vi "write_param.vi"   [LabVIEW 2012]
uses:
  FT_HMI.llb/GLOBAL_PUMPS_PARAMS.vi
  FT_HMI.llb/GLOBAL_GEN.vi
  ADS.llb/Global DIOs.vi
types:
  T1 = cluster{"VAC":cluster{"ENABLE":bool, "PUMPING_TIME [ms]":dbl, "MEASUREMENT_TIME [ms]":dbl, "PRESSURE_LIMIT [bar]":sgl}, "Q1":cluster{"ENABLE":bool, "PUMPING_TIME  [ms]":dbl, "MEASUREMENT_TIME  [ms]":sgl, "FLOW_TARGET  [ml/min]":sgl, "FLOW_LIMIT_UP  [ml/min]":sgl, "FLOW_LIMIT_DOWN [ml/min]":sgl, "PRESSURE_TARGET [bar]":sgl, "PRESSURE_LIMIT_UP [bar]":sgl, "PRESSURE_LIMIT_DOWN [bar]":sgl, "MAX_FLOW":bool}, "Q2":cluster{"ENABLE":bool, "PUMPING_TIME [ms]":dbl, "MEASUREMENT_TIME [ms]":dbl, "FLOW_TARGET [ml/min]":sgl, "FLOW_LIMIT_UP [ml/min]":sgl, "FLOW_LIMIT_DOWN [ml/min]":sgl, "PRESSURE_TARGET [bar]":sgl, "PRESSURE_LIMIT_UP [bar]":sgl, "PRESSURE_LIMIT_DOWN [bar]":sgl, "MAX_FLOW":bool}, "PMAX":cluster{"ENABLE":bool, "PUMPING_TIME [ms]":dbl, "MEASUREMENT_TIME [ms]":dbl, "PRESSURE_LIMIT [bar]":sgl, "PRESSURE_LOOSE_TIME [ms]":sgl}, "PRINT":cluster{"ENABLE":bool}, "SUPPLY":cluster{"VOLTAGE [V]":dbl, "FREQUENCY [Hz]":dbl}}
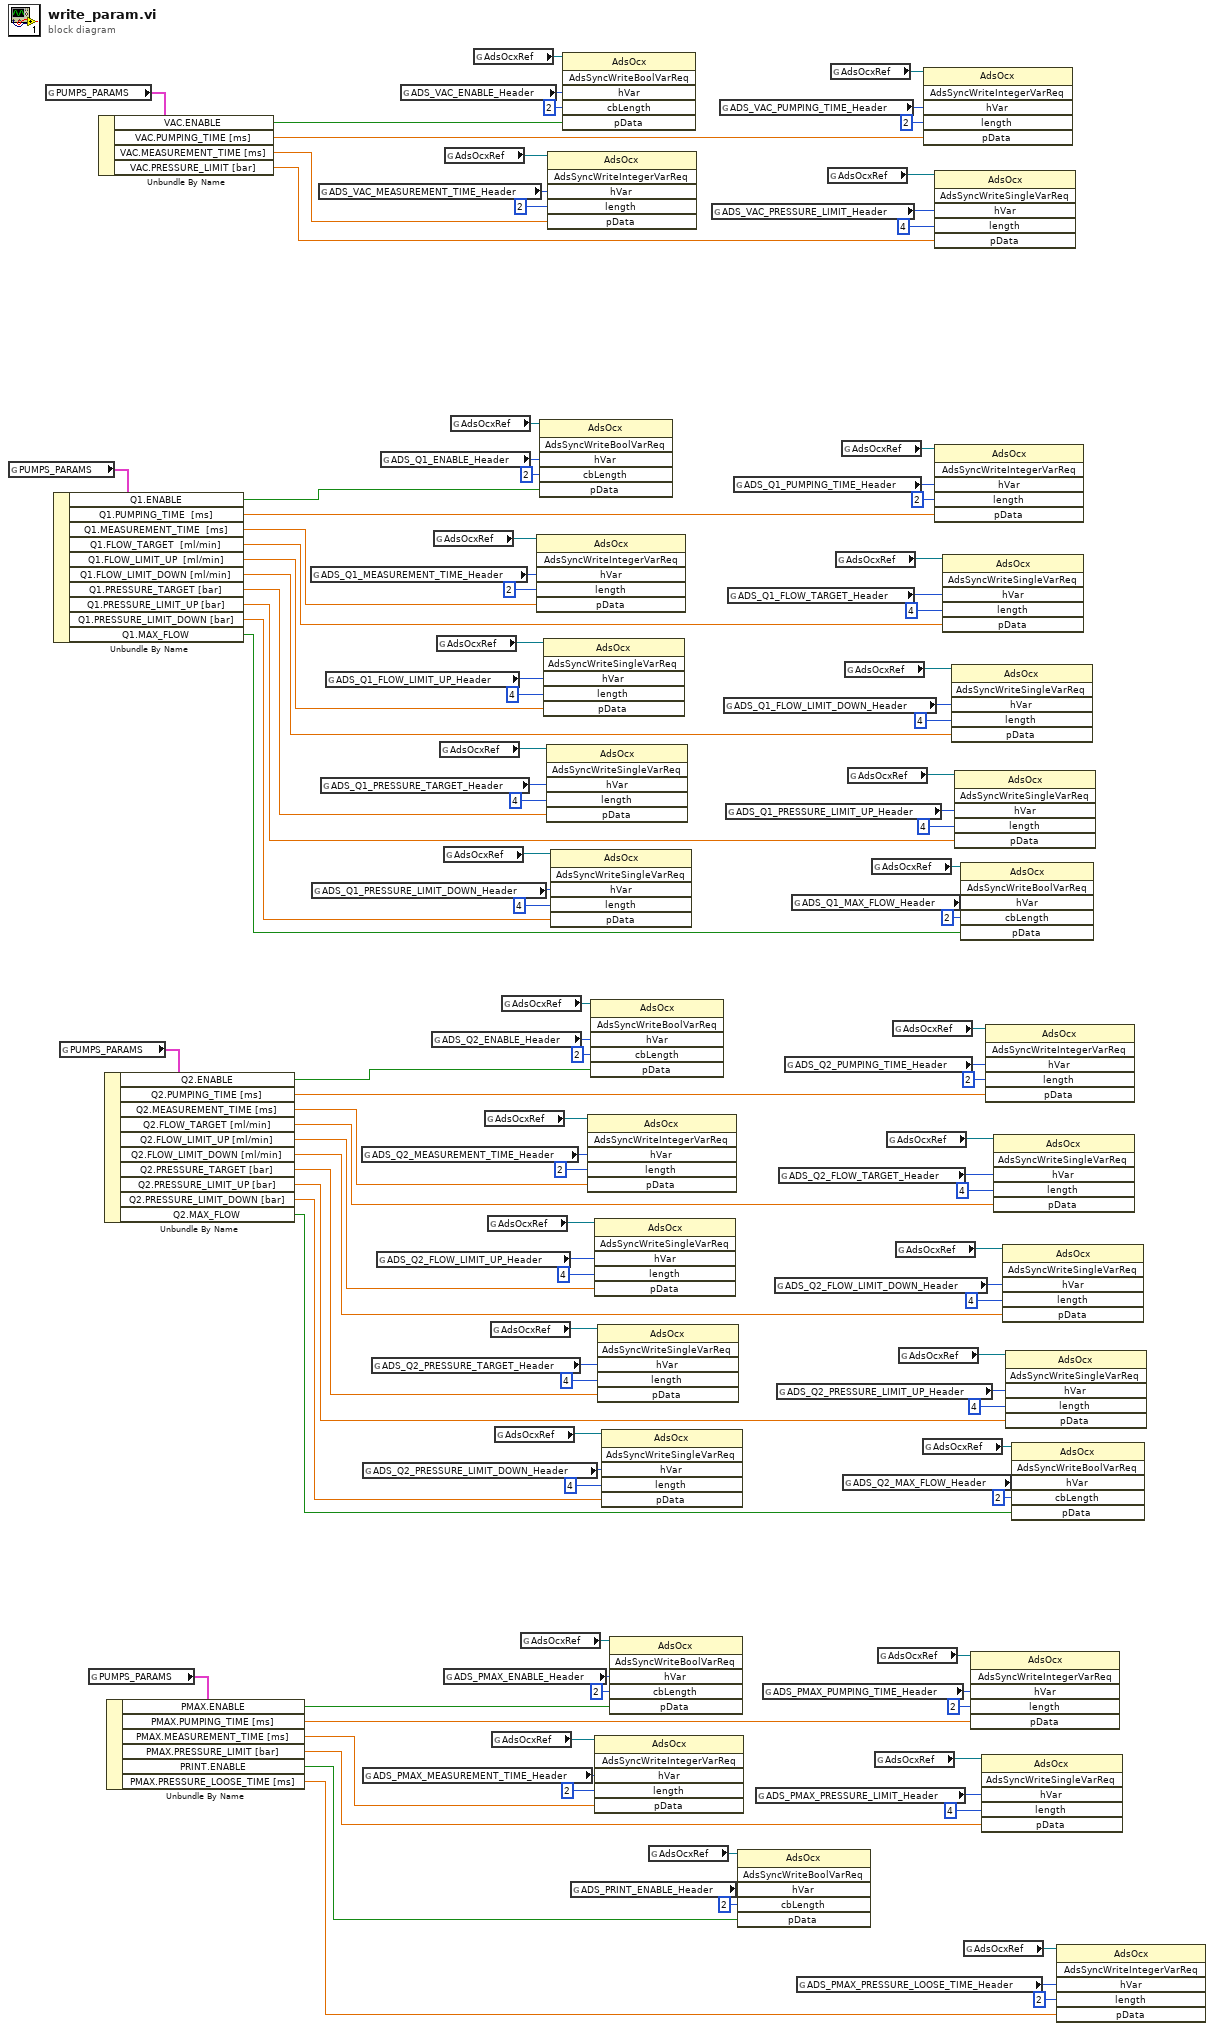
[diagram p0: block diagram]
diagram:
  n1 = global read "GLOBAL_PUMPS_PARAMS.vi" "PUMPS_PARAMS"() -> (w107:T1)
  n2 = global read "GLOBAL_PUMPS_PARAMS.vi" "PUMPS_PARAMS"() -> (w124:T1)
  n3 = Unbundle By Name(w107) -> ("Q1.ENABLE"=w103:bool, "Q1.PUMPING_TIME  [ms]"=w99:dbl, "Q1.MEASUREMENT_TIME  [ms]"=w95:sgl, "Q1.FLOW_TARGET  [ml/min]"=w91:sgl, "Q1.FLOW_LIMIT_UP  [ml/min]"=w83:sgl, "Q1.FLOW_LIMIT_DOWN [ml/min]"=w84:sgl, "Q1.PRESSURE_TARGET [bar]"=w76:sgl, "Q1.PRESSURE_LIMIT_UP [bar]"=w75:sgl, "Q1.PRESSURE_LIMIT_DOWN [bar]"=w71:sgl, "Q1.MAX_FLOW"=w67:bool)
  n4 = global read "GLOBAL_PUMPS_PARAMS.vi" "PUMPS_PARAMS"() -> (w66:T1)
  n5 = global read "GLOBAL_PUMPS_PARAMS.vi" "PUMPS_PARAMS"() -> (w25:T1)
  n6 = Unbundle By Name(w124) -> ("VAC.ENABLE"=w120:bool, "VAC.PUMPING_TIME [ms]"=w116:dbl, "VAC.MEASUREMENT_TIME [ms]"=w112:dbl, "VAC.PRESSURE_LIMIT [bar]"=w108:sgl)
  n7 = Unbundle By Name(w66) -> ("Q2.ENABLE"=w62:bool, "Q2.PUMPING_TIME [ms]"=w58:dbl, "Q2.MEASUREMENT_TIME [ms]"=w54:dbl, "Q2.FLOW_TARGET [ml/min]"=w50:sgl, "Q2.FLOW_LIMIT_UP [ml/min]"=w42:sgl, "Q2.FLOW_LIMIT_DOWN [ml/min]"=w43:sgl, "Q2.PRESSURE_TARGET [bar]"=w35:sgl, "Q2.PRESSURE_LIMIT_UP [bar]"=w34:sgl, "Q2.PRESSURE_LIMIT_DOWN [bar]"=w30:sgl, "Q2.MAX_FLOW"=w26:bool)
  n8 = Unbundle By Name(w25) -> ("PMAX.ENABLE"=w21:bool, "PMAX.PUMPING_TIME [ms]"=w17:dbl, "PMAX.MEASUREMENT_TIME [ms]"=w13:dbl, "PMAX.PRESSURE_LIMIT [bar]"=w9:sgl, "PRINT.ENABLE"=w5:bool, "PMAX.PRESSURE_LOOSE_TIME [ms]"=w1:sgl)
  n9 = global read "Global DIOs.vi" "ADS_Q1_MEASUREMENT_TIME_Header"() -> (w96:i32)
  n10 = global read "Global DIOs.vi" "ADS_Q1_PRESSURE_LIMIT_DOWN_Header"() -> (w72:i32)
  n11 = global read "Global DIOs.vi" "ADS_VAC_MEASUREMENT_TIME_Header"() -> (w113:i32)
  n12 = global read "Global DIOs.vi" "ADS_Q1_PRESSURE_TARGET_Header"() -> (w80:i32)
  n13 = global read "Global DIOs.vi" "ADS_Q1_FLOW_LIMIT_UP_Header"() -> (w88:i32)
  n14 = global read "Global DIOs.vi" "ADS_Q2_MEASUREMENT_TIME_Header"() -> (w55:i32)
  n15 = global read "Global DIOs.vi" "ADS_Q2_PRESSURE_LIMIT_DOWN_Header"() -> (w31:i32)
  n16 = global read "Global DIOs.vi" "ADS_PMAX_MEASUREMENT_TIME_Header"() -> (w14:i32)
  n17 = global read "Global DIOs.vi" "ADS_Q2_PRESSURE_TARGET_Header"() -> (w39:i32)
  n18 = global read "Global DIOs.vi" "ADS_Q2_FLOW_LIMIT_UP_Header"() -> (w47:i32)
  n19 = global read "Global DIOs.vi" "ADS_Q1_ENABLE_Header"() -> (w104:i32)
  n20 = global read "Global DIOs.vi" "ADS_VAC_ENABLE_Header"() -> (w121:i32)
  n21 = global read "Global DIOs.vi" "ADS_Q2_ENABLE_Header"() -> (w63:i32)
  n22 = global read "GLOBAL_GEN.vi" "AdsOcxRef"() -> (w97:refnum<k7>)
  n23 = global read "GLOBAL_GEN.vi" "AdsOcxRef"() -> (w89:refnum<k7>)
  n24 = global read "GLOBAL_GEN.vi" "AdsOcxRef"() -> (w81:refnum<k7>)
  n25 = global read "GLOBAL_GEN.vi" "AdsOcxRef"() -> (w73:refnum<k7>)
  n26 = global read "Global DIOs.vi" "ADS_PMAX_ENABLE_Header"() -> (w22:i32)
  n27 = global read "GLOBAL_GEN.vi" "AdsOcxRef"() -> (w114:refnum<k7>)
  n28 = global read "GLOBAL_GEN.vi" "AdsOcxRef"() -> (w105:refnum<k7>)
  n29 = global read "GLOBAL_GEN.vi" "AdsOcxRef"() -> (w122:refnum<k7>)
  n30 = global read "GLOBAL_GEN.vi" "AdsOcxRef"() -> (w56:refnum<k7>)
  n31 = global read "GLOBAL_GEN.vi" "AdsOcxRef"() -> (w48:refnum<k7>)
  n32 = global read "GLOBAL_GEN.vi" "AdsOcxRef"() -> (w40:refnum<k7>)
  n33 = global read "GLOBAL_GEN.vi" "AdsOcxRef"() -> (w15:refnum<k7>)
  n34 = global read "GLOBAL_GEN.vi" "AdsOcxRef"() -> (w32:refnum<k7>)
  n35 = global read "GLOBAL_GEN.vi" "AdsOcxRef"() -> (w64:refnum<k7>)
  n36 = global read "GLOBAL_GEN.vi" "AdsOcxRef"() -> (w23:refnum<k7>)
  n37 = invoke class="AdsOcx" method="AdsSyncWriteIntegerVarReq"(reference=w97, "hVar"=w96, "length"=2 ("phConnect"), "pData"=w95) -> ()  [unwired: 2 in, 6 out]
  n38 = invoke class="AdsOcx" method="AdsSyncWriteBoolVarReq"(reference=w105, "hVar"=w104, "cbLength"=2 ("phConnect"), "pData"=w103) -> ()  [unwired: 2 in, 6 out]
  n39 = invoke class="AdsOcx" method="AdsSyncWriteSingleVarReq"(reference=w89, "hVar"=w88, "length"=4 ("phConnect"), "pData"=w83) -> ()  [unwired: 2 in, 6 out]
  n40 = invoke class="AdsOcx" method="AdsSyncWriteSingleVarReq"(reference=w81, "hVar"=w80, "length"=4 ("phConnect"), "pData"=w76) -> ()  [unwired: 2 in, 6 out]
  n41 = invoke class="AdsOcx" method="AdsSyncWriteIntegerVarReq"(reference=w114, "hVar"=w113, "length"=2 ("phConnect"), "pData"=w112) -> ()  [unwired: 2 in, 6 out]
  n42 = invoke class="AdsOcx" method="AdsSyncWriteSingleVarReq"(reference=w73, "hVar"=w72, "length"=4 ("phConnect"), "pData"=w71) -> ()  [unwired: 2 in, 6 out]
  n43 = invoke class="AdsOcx" method="AdsSyncWriteBoolVarReq"(reference=w122, "hVar"=w121, "cbLength"=2 ("phConnect"), "pData"=w120) -> ()  [unwired: 2 in, 6 out]
  n44 = global read "Global DIOs.vi" "ADS_PRINT_ENABLE_Header"() -> (w6:i32)
  n45 = invoke class="AdsOcx" method="AdsSyncWriteIntegerVarReq"(reference=w56, "hVar"=w55, "length"=2 ("phConnect"), "pData"=w54) -> ()  [unwired: 2 in, 6 out]
  n46 = invoke class="AdsOcx" method="AdsSyncWriteBoolVarReq"(reference=w64, "hVar"=w63, "cbLength"=2 ("phConnect"), "pData"=w62) -> ()  [unwired: 2 in, 6 out]
  n47 = invoke class="AdsOcx" method="AdsSyncWriteSingleVarReq"(reference=w48, "hVar"=w47, "length"=4 ("phConnect"), "pData"=w42) -> ()  [unwired: 2 in, 6 out]
  n48 = invoke class="AdsOcx" method="AdsSyncWriteIntegerVarReq"(reference=w15, "hVar"=w14, "length"=2 ("phConnect"), "pData"=w13) -> ()  [unwired: 2 in, 6 out]
  n49 = invoke class="AdsOcx" method="AdsSyncWriteSingleVarReq"(reference=w40, "hVar"=w39, "length"=4 ("phConnect"), "pData"=w35) -> ()  [unwired: 2 in, 6 out]
  n50 = invoke class="AdsOcx" method="AdsSyncWriteSingleVarReq"(reference=w32, "hVar"=w31, "length"=4 ("phConnect"), "pData"=w30) -> ()  [unwired: 2 in, 6 out]
  n51 = invoke class="AdsOcx" method="AdsSyncWriteBoolVarReq"(reference=w23, "hVar"=w22, "cbLength"=2 ("phConnect"), "pData"=w21) -> ()  [unwired: 2 in, 6 out]
  n52 = global read "GLOBAL_GEN.vi" "AdsOcxRef"() -> (w7:refnum<k7>)
  n53 = global read "Global DIOs.vi" "ADS_VAC_PRESSURE_LIMIT_Header"() -> (w109:i32)
  n54 = global read "Global DIOs.vi" "ADS_VAC_PUMPING_TIME_Header"() -> (w117:i32)
  n55 = global read "Global DIOs.vi" "ADS_Q1_FLOW_LIMIT_DOWN_Header"() -> (w85:i32)
  n56 = global read "Global DIOs.vi" "ADS_Q1_PRESSURE_LIMIT_UP_Header"() -> (w77:i32)
  n57 = global read "Global DIOs.vi" "ADS_Q1_FLOW_TARGET_Header"() -> (w92:i32)
  n58 = global read "Global DIOs.vi" "ADS_Q1_PUMPING_TIME_Header"() -> (w100:i32)
  n59 = invoke class="AdsOcx" method="AdsSyncWriteBoolVarReq"(reference=w7, "hVar"=w6, "cbLength"=2 ("phConnect"), "pData"=w5) -> ()  [unwired: 2 in, 6 out]
  n60 = global read "Global DIOs.vi" "ADS_PMAX_PRESSURE_LIMIT_Header"() -> (w10:i32)
  n61 = global read "Global DIOs.vi" "ADS_PMAX_PUMPING_TIME_Header"() -> (w18:i32)
  n62 = global read "Global DIOs.vi" "ADS_Q2_FLOW_LIMIT_DOWN_Header"() -> (w44:i32)
  n63 = global read "Global DIOs.vi" "ADS_Q2_PRESSURE_LIMIT_UP_Header"() -> (w36:i32)
  n64 = global read "Global DIOs.vi" "ADS_Q2_FLOW_TARGET_Header"() -> (w51:i32)
  n65 = global read "Global DIOs.vi" "ADS_Q2_PUMPING_TIME_Header"() -> (w59:i32)
  n66 = global read "Global DIOs.vi" "ADS_Q1_MAX_FLOW_Header"() -> (w68:i32)
  n67 = global read "Global DIOs.vi" "ADS_PMAX_PRESSURE_LOOSE_TIME_Header"() -> (w2:i32)
  n68 = global read "GLOBAL_GEN.vi" "AdsOcxRef"() -> (w110:refnum<k7>)
  n69 = global read "GLOBAL_GEN.vi" "AdsOcxRef"() -> (w118:refnum<k7>)
  n70 = global read "GLOBAL_GEN.vi" "AdsOcxRef"() -> (w93:refnum<k7>)
  n71 = global read "GLOBAL_GEN.vi" "AdsOcxRef"() -> (w101:refnum<k7>)
  n72 = global read "Global DIOs.vi" "ADS_Q2_MAX_FLOW_Header"() -> (w27:i32)
  n73 = global read "GLOBAL_GEN.vi" "AdsOcxRef"() -> (w86:refnum<k7>)
  n74 = global read "GLOBAL_GEN.vi" "AdsOcxRef"() -> (w78:refnum<k7>)
  n75 = global read "GLOBAL_GEN.vi" "AdsOcxRef"() -> (w69:refnum<k7>)
  n76 = global read "GLOBAL_GEN.vi" "AdsOcxRef"() -> (w11:refnum<k7>)
  n77 = global read "GLOBAL_GEN.vi" "AdsOcxRef"() -> (w19:refnum<k7>)
  n78 = global read "GLOBAL_GEN.vi" "AdsOcxRef"() -> (w52:refnum<k7>)
  n79 = global read "GLOBAL_GEN.vi" "AdsOcxRef"() -> (w60:refnum<k7>)
  n80 = global read "GLOBAL_GEN.vi" "AdsOcxRef"() -> (w45:refnum<k7>)
  n81 = global read "GLOBAL_GEN.vi" "AdsOcxRef"() -> (w37:refnum<k7>)
  n82 = global read "GLOBAL_GEN.vi" "AdsOcxRef"() -> (w28:refnum<k7>)
  n83 = invoke class="AdsOcx" method="AdsSyncWriteIntegerVarReq"(reference=w118, "hVar"=w117, "length"=2 ("phConnect"), "pData"=w116) -> ()  [unwired: 2 in, 6 out]
  n84 = invoke class="AdsOcx" method="AdsSyncWriteSingleVarReq"(reference=w110, "hVar"=w109, "length"=4 ("phConnect"), "pData"=w108) -> ()  [unwired: 2 in, 6 out]
  n85 = invoke class="AdsOcx" method="AdsSyncWriteIntegerVarReq"(reference=w101, "hVar"=w100, "length"=2 ("phConnect"), "pData"=w99) -> ()  [unwired: 2 in, 6 out]
  n86 = invoke class="AdsOcx" method="AdsSyncWriteSingleVarReq"(reference=w93, "hVar"=w92, "length"=4 ("phConnect"), "pData"=w91) -> ()  [unwired: 2 in, 6 out]
  n87 = invoke class="AdsOcx" method="AdsSyncWriteSingleVarReq"(reference=w86, "hVar"=w85, "length"=4 ("phConnect"), "pData"=w84) -> ()  [unwired: 2 in, 6 out]
  n88 = invoke class="AdsOcx" method="AdsSyncWriteSingleVarReq"(reference=w78, "hVar"=w77, "length"=4 ("phConnect"), "pData"=w75) -> ()  [unwired: 2 in, 6 out]
  n89 = invoke class="AdsOcx" method="AdsSyncWriteBoolVarReq"(reference=w69, "hVar"=w68, "cbLength"=2 ("phConnect"), "pData"=w67) -> ()  [unwired: 2 in, 6 out]
  n90 = global read "GLOBAL_GEN.vi" "AdsOcxRef"() -> (w3:refnum<k7>)
  n91 = invoke class="AdsOcx" method="AdsSyncWriteIntegerVarReq"(reference=w19, "hVar"=w18, "length"=2 ("phConnect"), "pData"=w17) -> ()  [unwired: 2 in, 6 out]
  n92 = invoke class="AdsOcx" method="AdsSyncWriteSingleVarReq"(reference=w11, "hVar"=w10, "length"=4 ("phConnect"), "pData"=w9) -> ()  [unwired: 2 in, 6 out]
  n93 = invoke class="AdsOcx" method="AdsSyncWriteIntegerVarReq"(reference=w60, "hVar"=w59, "length"=2 ("phConnect"), "pData"=w58) -> ()  [unwired: 2 in, 6 out]
  n94 = invoke class="AdsOcx" method="AdsSyncWriteSingleVarReq"(reference=w52, "hVar"=w51, "length"=4 ("phConnect"), "pData"=w50) -> ()  [unwired: 2 in, 6 out]
  n95 = invoke class="AdsOcx" method="AdsSyncWriteSingleVarReq"(reference=w45, "hVar"=w44, "length"=4 ("phConnect"), "pData"=w43) -> ()  [unwired: 2 in, 6 out]
  n96 = invoke class="AdsOcx" method="AdsSyncWriteSingleVarReq"(reference=w37, "hVar"=w36, "length"=4 ("phConnect"), "pData"=w34) -> ()  [unwired: 2 in, 6 out]
  n97 = invoke class="AdsOcx" method="AdsSyncWriteBoolVarReq"(reference=w28, "hVar"=w27, "cbLength"=2 ("phConnect"), "pData"=w26) -> ()  [unwired: 2 in, 6 out]
  n98 = invoke class="AdsOcx" method="AdsSyncWriteIntegerVarReq"(reference=w3, "hVar"=w2, "length"=2 ("phConnect"), "pData"=w1) -> ()  [unwired: 2 in, 6 out]
